vi "IV.vi"() -> ()   [LabVIEW 2021]
uses:
  Libraries/Instruments/Controls/IV Config.ctl
  Libraries/Instruments/SRS/CS580 Driver/CS580 Driver.lvclass
  C:/Git/NHMFL_Core/Libraries/Instruments/VISA Instrument/VISA Instrument.lvclass
  C:/Git/NHMFL_Core/Libraries/Instruments/Instrument Driver/Instrument Driver.lvclass
  Libraries/Instruments/EG_G/Signal Recovery Driver/Signal Recovery Driver.lvclass
  IV.lvclass
  Libraries/Instruments/VISA Instrument/VISA Instrument.lvclass/VISA Instrument.ctl
  Libraries/Instruments/Instrument Driver/Instrument Driver.lvclass/Instrument Driver.ctl
  Libraries/Instruments/VISA Instrument/Write VISA resource.vi
  Libraries/Instruments/Instrument Driver/Write Recorder name.vi
panel:
  out "File Path":path
  out "XY Graph":cluster{dbl[], dbl[]}[](graph)
  in  "Lockin VISA":refnum<visa-resource-name>="GPIB0::11::INSTR"
  in  "Current source VISA":refnum<visa-resource-name>="COM5"
  in  "Configuration":T1={"Start current"=-0.0005, "End current"=0.0005, "Current step"=1e-05, "Step time"=5.0} {"Step time" format="%#_6ps"; "Current step" format="%#_6pA"; "End current" format="%#_6pA"; "Start current" format="%#_6pA"}
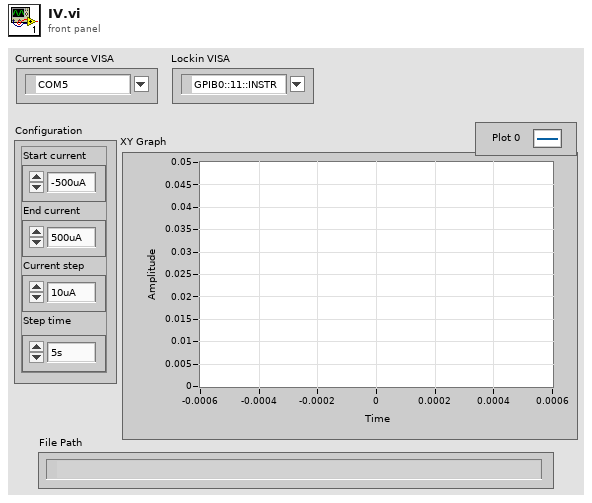
[diagram p1: front panel]
types:
  T1 = typedef "IV Config.ctl" = cluster{"Start current":dbl, "End current":dbl, "Current step":dbl, "Step time":dbl}
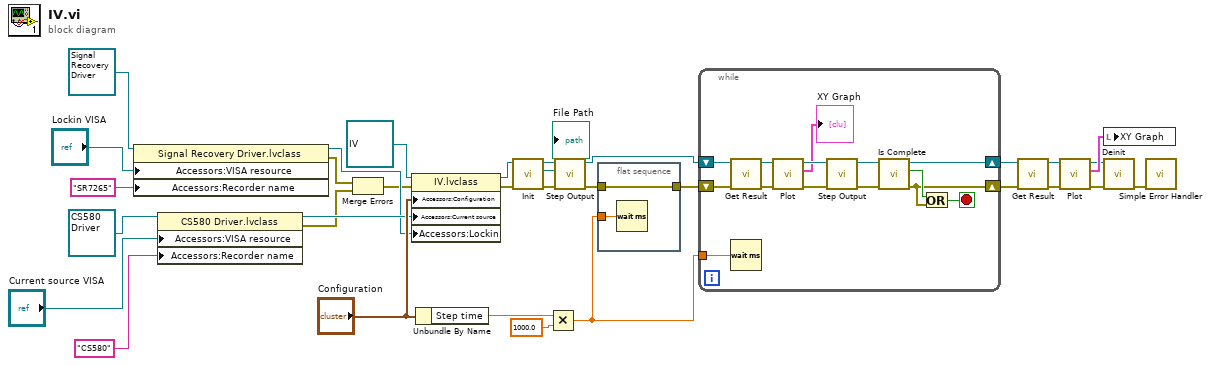
[diagram p0: block diagram]
diagram:
  n1 = property class="Signal Recovery Driver.lvclass"(reference=refnum<class "Signal Recovery Driver.lvclass"> refnum ("Signal Recovery Driver in"), "Accessors:VISA resource"="Lockin VISA", "Accessors:Recorder name"="SR7265" ("Recorder name")) -> (reference out=w21:refnum<class "Signal Recovery Driver.lvclass">, error out=w25:errorcluster)  [unwired: 1 in]
  n2 = property class="CS580 Driver.lvclass"(reference=refnum<class "CS580 Driver.lvclass"> refnum ("CS580 Driver in"), "Accessors:VISA resource"="Current source VISA", "Accessors:Recorder name"="CS580" ("Recorder name")) -> (reference out=w22:refnum<class "CS580 Driver.lvclass">, error out=w12:errorcluster)  [unwired: 1 in]
  n3 = Merge Errors(w25, w12) -> (w20:errorcluster)
  n4 = property class="IV.lvclass"(reference=refnum<class "IV.lvclass"> refnum ("IV.lvclass"), error in=w20, "Accessors:Configuration"="Configuration", "Accessors:Current source "=w22, "Accessors:Lockin"=w21) -> (reference out=w17:refnum<class "IV.lvclass">, error out=w16:errorcluster)
  n5 = Unbundle By Name("Configuration") -> ("Step time"=w30:dbl)
  n6 = call-dynamic "Init.vi"("error in (no error)"=w16, "IV in"=w17) -> ("error out"=w19:errorcluster, "File Path"=→"File Path":path, "IV out"=w18:refnum<class "IV.lvclass">)  [unwired: 7 in]
  n7 = Multiply(x=w30, y=1000.0) -> (x*y=w28:dbl)
  n8 = call-dynamic "Step Output.vi"("error in (no error)"=w19, "IV in"=w18) -> ("error out"=w15:errorcluster, "IV out"=w13:refnum<class "IV.lvclass">)  [unwired: 8 in]
  n9 = flat-sequence {
    tunnel: w28 -> [w34]
    tunnel: w15 -> [w33]
    tunnel: [w33] -> w14
    frame #0 {
      n10 = Wait (ms)(milliseconds to wait=w34) -> ()  [unwired: 1 out]
    }
  }
  n11 = while {
    shift-right: [w36] -> w11
    shift-left: w14 -> [w46]
    tunnel: w28 -> [w48]
    shift-right: [w43] -> w10
    shift-left: w13 -> [w47]
    stop <- w35 stop-if-true
    n12 = call-dynamic "Get Result.vi"("error in (no error)"=w46, "IV in"=w47) -> ("error out"=w41:errorcluster, "IV out"=w42:refnum<class "IV.lvclass">)  [unwired: 6 in, 2 out]
    n13 = Wait (ms)(milliseconds to wait=w48) -> ()  [unwired: 1 out]
    n14 = call-dynamic "Plot.vi"("error in (no error)"=w41, "IV in"=w42) -> ("error out"=w39:errorcluster, "Plot"=→"XY Graph":cluster{dbl[], dbl[]}[], "IV out"=w40:refnum<class "IV.lvclass">)  [unwired: 7 in]
    n15 = call-dynamic "Step Output.vi"("error in (no error)"=w39, "IV in"=w40) -> ("error out"=w44:errorcluster, "IV out"=w45:refnum<class "IV.lvclass">)  [unwired: 8 in]
    n16 = call-dynamic "Is Complete.vi"("error in (no error)"=w44, "IV in"=w45) -> ("error out"=w36:errorcluster, "Is complete?"=w37:bool, "IV out"=w43:refnum<class "IV.lvclass">)  [unwired: 7 in]
    n17 = Or(x=w37, y=w36) -> (x .or. y?=w35:bool)
  }
  n18 = call-dynamic "Get Result.vi"("error in (no error)"=w11, "IV in"=w10) -> ("error out"=w6:errorcluster, "IV out"=w7:refnum<class "IV.lvclass">)  [unwired: 6 in, 2 out]
  n19 = call-dynamic "Plot.vi"("error in (no error)"=w6, "IV in"=w7) -> ("error out"=w4:errorcluster, "Plot"=w5:cluster{dbl[], dbl[]}[], "IV out"=w3:refnum<class "IV.lvclass">)  [unwired: 7 in]
  n20 = local write "XY Graph"(w5) -> ()
  n21 = call-dynamic "Deinit.vi"("error in (no error)"=w4, "IV in"=w3) -> ("error out"=w2:errorcluster)  [unwired: 8 in, 1 out]
  n22 = call <vilib>:"Simple Error Handler.vi"("error in (no error)"=w2) -> ()  [unwired: 4 in, 5 out]
